vi "Write Handle.vi"(8 "error in (no error)":errorcluster, 10 "Handle":refnum<class "LoggingHandle.lvclass">, 11 "HandleHolder in":refnum<class "HandleHolder.lvclass">) -> (0 "error out":errorcluster, 3 "HandleHolder out":refnum<class "HandleHolder.lvclass">)   [LabVIEW 2024, in "HandleHolder.lvclass"]
uses:
  HandleHolder.lvclass
  LogHandle/Interface/LoggingHandle.lvclass
  HandleHolder.lvclass/HandleHolder.ctl
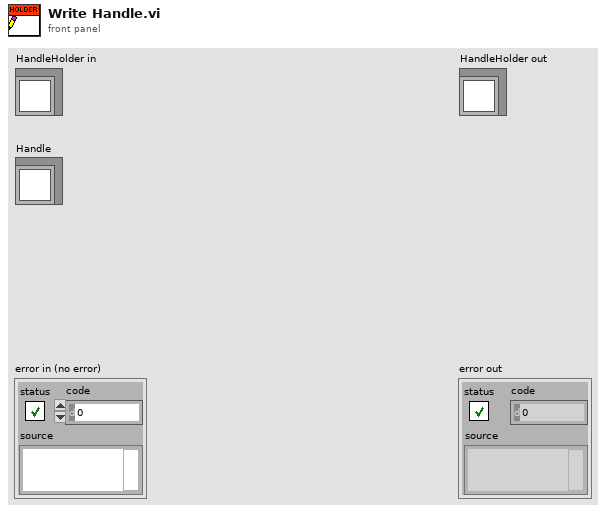
[diagram p1: front panel]
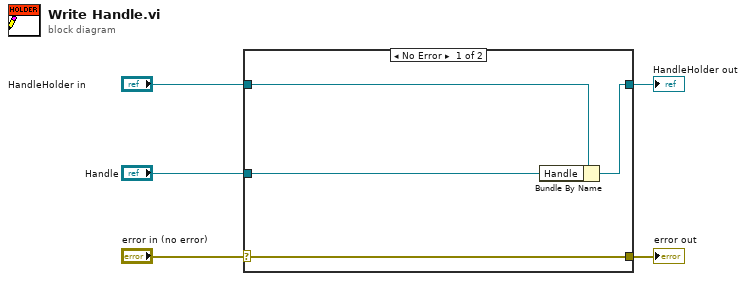
[diagram p0: block diagram]
diagram:
  n1 = case shown="No Error" "error in (no error)" {
    selector: "error in (no error)" -> [w9 w10]
    tunnel: [w9 w10] -> w4
    tunnel: [w7 w11] -> w2
    tunnel: "HandleHolder in" -> [w8 w11]
    tunnel: "Handle" -> [w6 _]
    frame No Error {
      n2 = Bundle By Name(cluster=w8, "Handle"=w6) -> (w7:refnum<class "HandleHolder.lvclass">)
    }
    frame Error {
    }
  }
  "error out" <- w4
  "HandleHolder out" <- w2
